vi "current version.vi"() -> ()   [LabVIEW 2013, in "Shared Library Module configuration.lvclass"]
doc: "#CodeRequired\nThis global variable stores the current version of the module and should be updated as serialization formats change.Platypus Framework 1.0.1.60\nNI Systems Engineering - National Instruments"
uses:
  Shared Library Module configuration.lvclass
panel:
  out "current version":string="1.0.0.0"
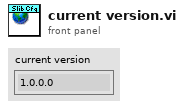
[diagram p1: front panel]
diagram:
